vi "LM3Sxxxx_Timer_Config.vi"(8 "error in (no error)":errorcluster, 10 "Config Data":string[](array[string]), 11 "Interrupt Name":string) -> (0 "error out":errorcluster, 3 "Interrupt Configuration":string[](array[string]))   [LabVIEW 2011]
panel:
  in  "Trigger":u32(ring) items=["Rising edge"=0, "Falling edge"=1028, "Both edges"=3084]
  in  "Trigger":u32(ring) items=["Rising edge"=0, "Falling edge"=1028]
  in  "Units":u32(ring)=1 items=["Milliseconds"=1, "Microseconds"=2, "Ticks"=0]
  in  "Count":u16=1000
  in  "Count":u16=1000
  in  "Period":u32=1000
  in  "edge capture":bool
  in  "timer capture":bool
  in  "timer":bool=TRUE
  in  "help":bool
  in  "cancel":bool
  in  "ok":bool
  # "Mode"
  # "32-bit Timer"
  # "16-bit Timer Capture"
  # "16-bit Edge Counter"
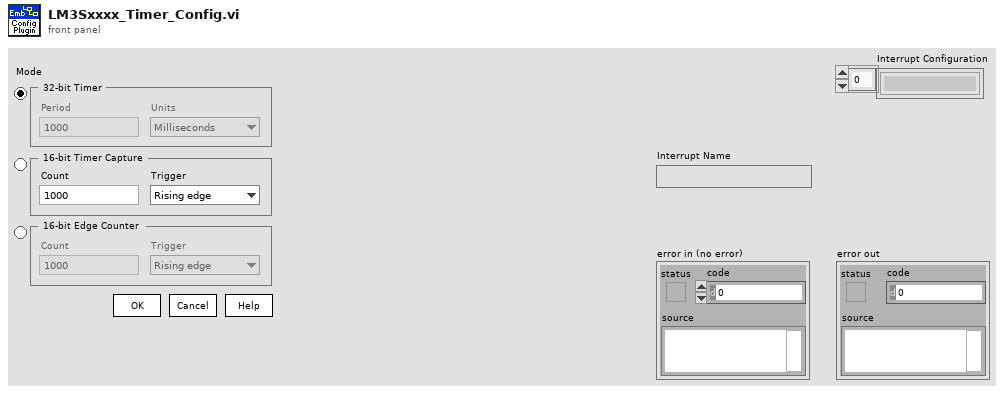
[diagram p1: front panel]
types:
  T1 = enum8{"Enabled", "Disabled", "Disabled and Grayed Out"}
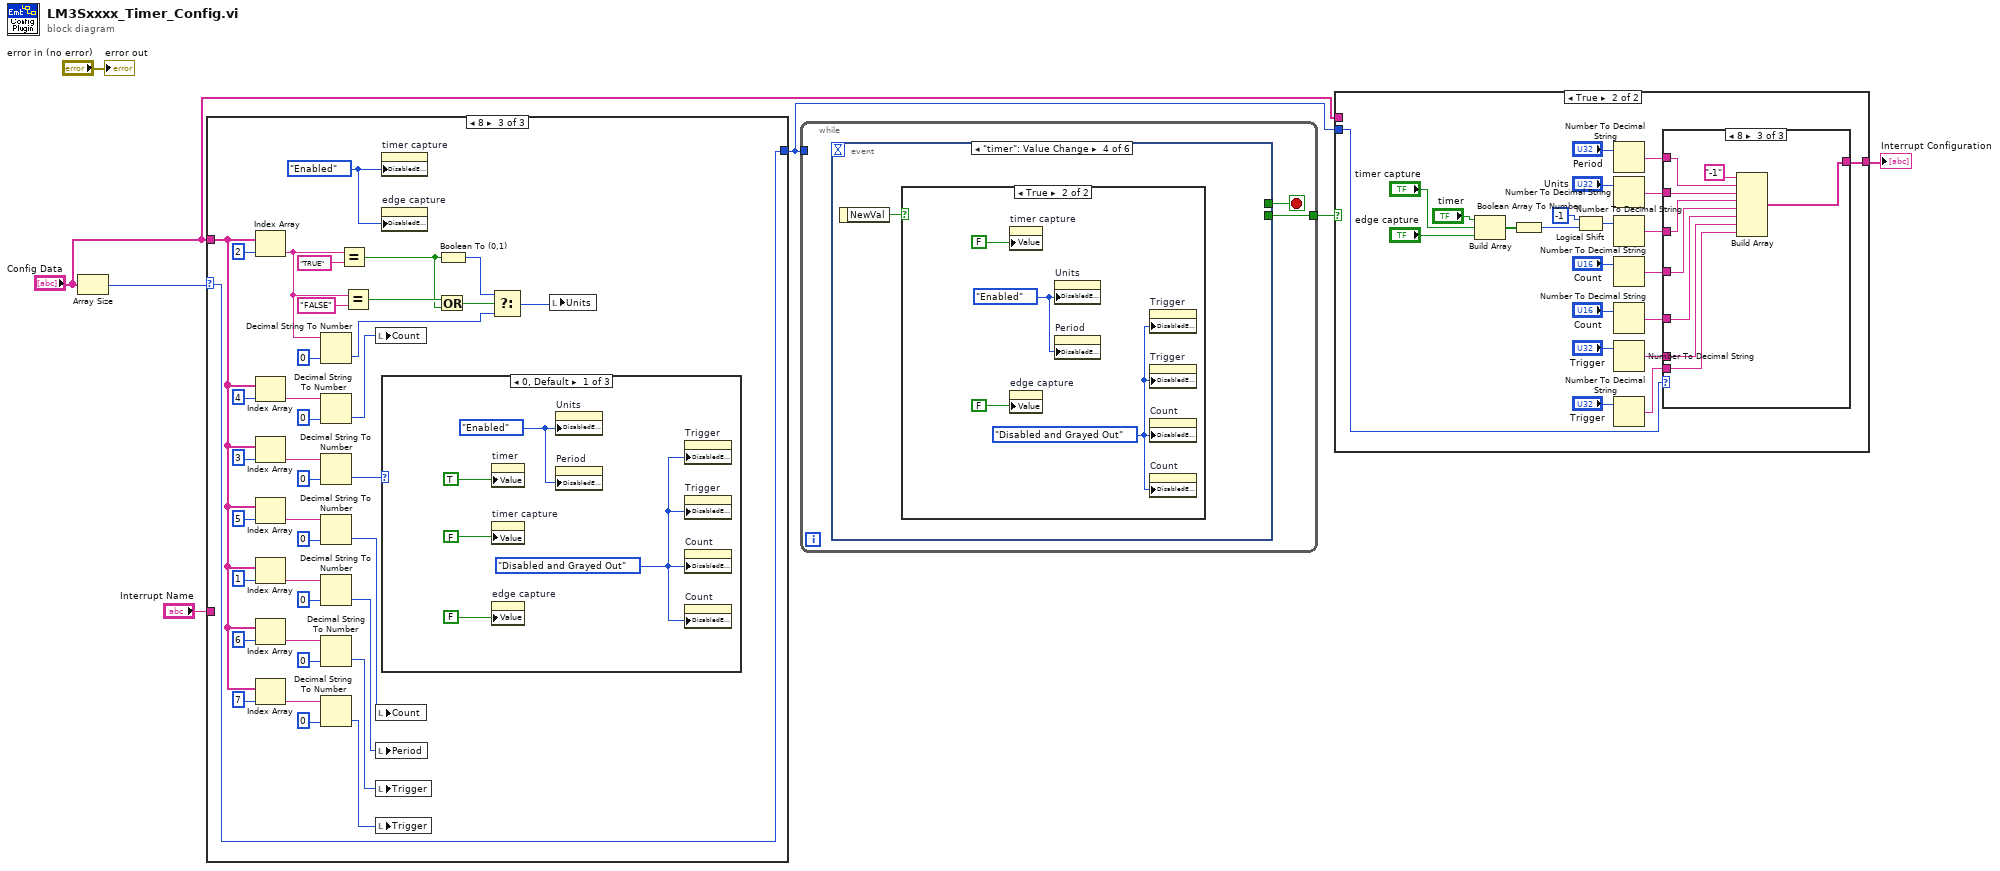
[diagram p0: block diagram]
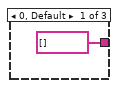
[diagram p3: hidden frame]
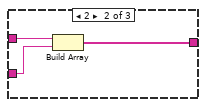
[diagram p4: hidden frame]
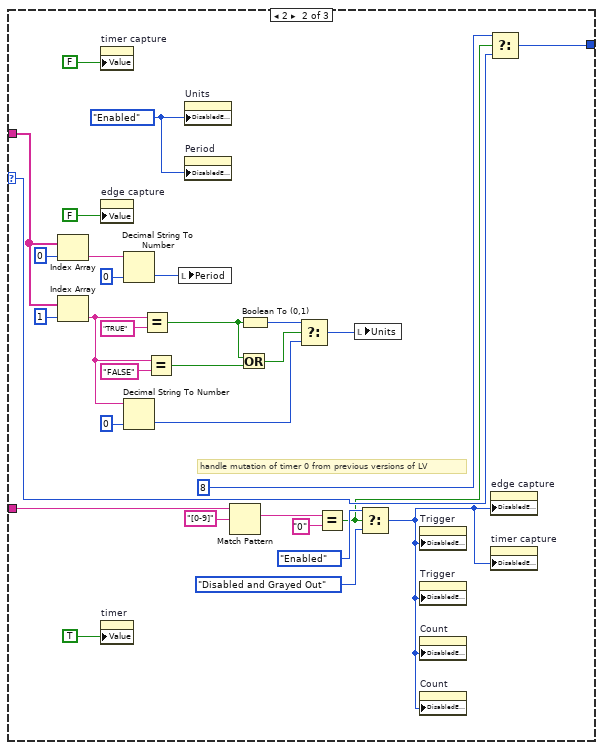
[diagram p6: hidden frame]
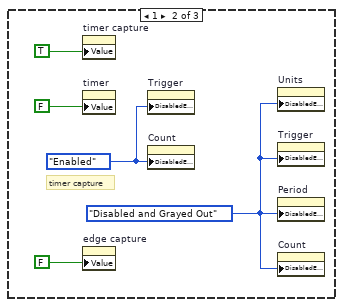
[diagram p7: hidden frame]
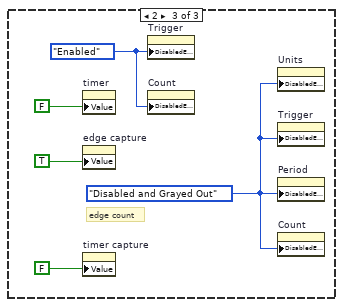
[diagram p8: hidden frame]
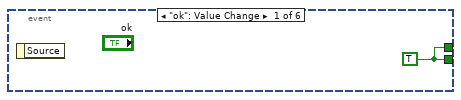
[diagram p9: hidden frame]
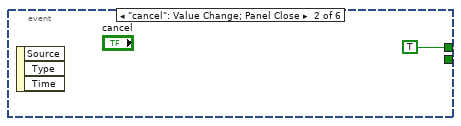
[diagram p10: hidden frame]
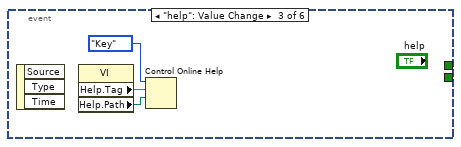
[diagram p11: hidden frame]
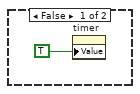
[diagram p12: hidden frame]
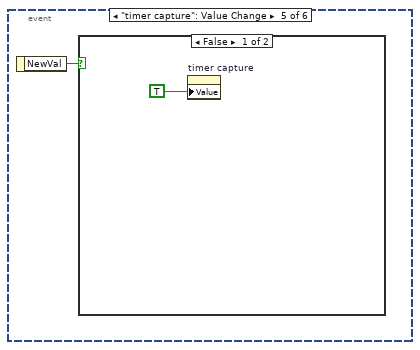
[diagram p13: hidden frame]
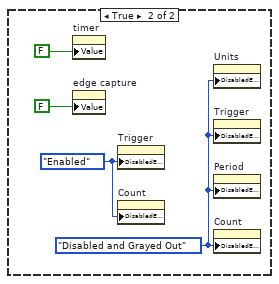
[diagram p14: hidden frame]
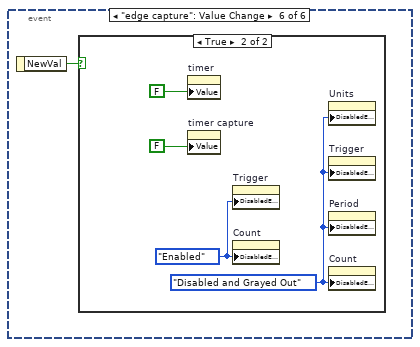
[diagram p15: hidden frame]
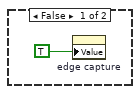
[diagram p16: hidden frame]
diagram:
  n1 = Array Size(array="Config Data") -> (size(s)=w3:i32)
  n2 = case shown="8" w3 {
    selector: w3 -> [w8 w23 w77]
    tunnel: "Config Data" -> [_ w39 w62]
    tunnel: [w8 w22 w77] -> w1
    tunnel: "Interrupt Name" -> [_ w27 _]
    frame Default {
    }
    frame 2 {
      w29 = T1."Enabled" ("Disabled")
      # "handle mutation of timer 0 from previous versions of LV"
      n3 = Index Array(array=w39, index=0) -> (element=w35:string)
      n4 = Index Array(array=w39, index=1) -> (element=w15:string)
      n5 = property on="timer capture" class="Bool (strict)"("Value"=FALSE ("timer capture")) -> ()  [unwired: 2 in, 2 out]
      n6 = property on="edge capture" class="Bool (strict)"("Value"=FALSE ("edge capture")) -> ()  [unwired: 2 in, 2 out]
      n7 = property on="timer" class="Bool (strict)"("Value"=TRUE ("timer")) -> ()  [unwired: 2 in, 2 out]
      n8 = Decimal String To Number(string=w35, default (0L)=u32 0) -> (number=w34:u32)  [unwired: 1 in, 1 out]
      n9 = Decimal String To Number(string=w15, default (0L)=u32 0) -> (number=w11:u32)  [unwired: 1 in, 1 out]
      n10 = Equal?(x=w15, y="TRUE") -> (x = y?=w14:bool)
      n11 = Equal?(x=w15, y="FALSE") -> (x = y?=w13:bool)
      n12 = local write "Period"(w34) -> ()
      n13 = property on="Units" class="Ring (strict)"("DisabledEnum"=w29) -> ()  [unwired: 2 in, 2 out]
      n14 = property on="Period" class="DigNum (strict)"("DisabledEnum"=w29) -> ()  [unwired: 2 in, 2 out]
      n15 = Match Pattern(string=w27, regular expression="[0-9]") -> (match substring=w20:string)  [unwired: 1 in, 3 out]
      n16 = Or(x=w14, y=w13) -> (x .or. y?=w12:bool)
      n17 = Boolean To (0,1)(Boolean=w14) -> (0, 1=w10:i16)
      n18 = Select(t=w10, s=w12, f=w11) -> (s? t:f=w9:u32)
      n19 = Equal?(x=w20, y="0") -> (x = y?=w19:bool)
      n20 = local write "Units"(w9) -> ()
      n21 = Select(t=T1."Enabled", s=w19, f=T1."Disabled and Grayed Out" ("Disabled")) -> (s? t:f=w25:T1)
      n22 = property on="Trigger" class="Ring (strict)"("DisabledEnum"=w25) -> ()  [unwired: 2 in, 2 out]
      n23 = property on="Trigger" class="Ring (strict)"("DisabledEnum"=w25) -> ()  [unwired: 2 in, 2 out]
      n24 = property on="Count" class="DigNum (strict)"("DisabledEnum"=w25) -> ()  [unwired: 2 in, 2 out]
      n25 = property on="Count" class="DigNum (strict)"("DisabledEnum"=w25) -> ()  [unwired: 2 in, 2 out]
      n26 = Select(t=8, s=w19, f=w23) -> (s? t:f=w22:i32)
      n27 = property on="edge capture" class="Bool (strict)"("DisabledEnum"=w25) -> ()  [unwired: 2 in, 2 out]
      n28 = property on="timer capture" class="Bool (strict)"("DisabledEnum"=w25) -> ()  [unwired: 2 in, 2 out]
    }
    frame 8 {
      w49 = T1."Enabled" ("Disabled")
      n29 = Index Array(array=w62, index=2) -> (element=w44:string)
      n30 = Index Array(array=w62, index=4) -> (element=w60:string)
      n31 = Index Array(array=w62, index=3) -> (element=w66:string)
      n32 = Index Array(array=w62, index=5) -> (element=w57:string)
      n33 = Index Array(array=w62, index=1) -> (element=w75:string)
      n34 = Index Array(array=w62, index=6) -> (element=w53:string)
      n35 = Index Array(array=w62, index=7) -> (element=w52:string)
      n36 = Decimal String To Number(string=w44, default (0L)=u32 0) -> (number=w41:u32)  [unwired: 1 in, 1 out]
      n37 = Decimal String To Number(string=w60, default (0L)=u16 0) -> (number=w59:u16)  [unwired: 1 in, 1 out]
      n38 = Decimal String To Number(string=w66, default (0L)=u32 0) -> (number=w65:u32)  [unwired: 1 in, 1 out]
      n39 = Decimal String To Number(string=w57, default (0L)=u16 0) -> (number=w56:u16)  [unwired: 1 in, 1 out]
      n40 = Decimal String To Number(string=w75, default (0L)=u32 0) -> (number=w71:u32)  [unwired: 1 in, 1 out]
      n41 = Decimal String To Number(string=w53, default (0L)=u32 0) -> (number=w51:u32)  [unwired: 1 in, 1 out]
      n42 = Decimal String To Number(string=w52, default (0L)=u32 0) -> (number=w50:u32)  [unwired: 1 in, 1 out]
      n43 = Equal?(x=w44, y="TRUE") -> (x = y?=w46:bool)
      n44 = Equal?(x=w44, y="FALSE") -> (x = y?=w47:bool)
      n45 = local write "Count"(w59) -> ()
      n46 = local write "Count"(w56) -> ()
      n47 = local write "Period"(w71) -> ()
      n48 = local write "Trigger"(w51) -> ()
      n49 = local write "Trigger"(w50) -> ()
      n50 = property on="timer capture" class="Bool (strict)"("DisabledEnum"=w49) -> ()  [unwired: 2 in, 2 out]
      n51 = property on="edge capture" class="Bool (strict)"("DisabledEnum"=w49) -> ()  [unwired: 2 in, 2 out]
      n52 = case shown="0, Default" w65 {
        frame 0, Default {
          w78 = T1."Disabled and Grayed Out" ("Disabled")
          w79 = T1."Enabled" ("Disabled")
          n53 = property on="timer" class="Bool (strict)"("Value"=TRUE ("timer")) -> ()  [unwired: 2 in, 2 out]
          n54 = property on="timer capture" class="Bool (strict)"("Value"=FALSE ("timer capture")) -> ()  [unwired: 2 in, 2 out]
          n55 = property on="edge capture" class="Bool (strict)"("Value"=FALSE ("edge capture")) -> ()  [unwired: 2 in, 2 out]
          n56 = property on="Units" class="Ring (strict)"("DisabledEnum"=w79) -> ()  [unwired: 2 in, 2 out]
          n57 = property on="Period" class="DigNum (strict)"("DisabledEnum"=w79) -> ()  [unwired: 2 in, 2 out]
          n58 = property on="Trigger" class="Ring (strict)"("DisabledEnum"=w78) -> ()  [unwired: 2 in, 2 out]
          n59 = property on="Trigger" class="Ring (strict)"("DisabledEnum"=w78) -> ()  [unwired: 2 in, 2 out]
          n60 = property on="Count" class="DigNum (strict)"("DisabledEnum"=w78) -> ()  [unwired: 2 in, 2 out]
          n61 = property on="Count" class="DigNum (strict)"("DisabledEnum"=w78) -> ()  [unwired: 2 in, 2 out]
        }
        frame 1 {
          w84 = T1."Enabled" ("Disabled")
          w83 = T1."Disabled and Grayed Out" ("Disabled")
          # "timer capture"
          n62 = property on="timer capture" class="Bool (strict)"("Value"=TRUE ("timer capture")) -> ()  [unwired: 2 in, 2 out]
          n63 = property on="timer" class="Bool (strict)"("Value"=FALSE ("timer")) -> ()  [unwired: 2 in, 2 out]
          n64 = property on="edge capture" class="Bool (strict)"("Value"=FALSE ("edge capture")) -> ()  [unwired: 2 in, 2 out]
          n65 = property on="Trigger" class="Ring (strict)"("DisabledEnum"=w84) -> ()  [unwired: 2 in, 2 out]
          n66 = property on="Count" class="DigNum (strict)"("DisabledEnum"=w84) -> ()  [unwired: 2 in, 2 out]
          n67 = property on="Units" class="Ring (strict)"("DisabledEnum"=w83) -> ()  [unwired: 2 in, 2 out]
          n68 = property on="Trigger" class="Ring (strict)"("DisabledEnum"=w83) -> ()  [unwired: 2 in, 2 out]
          n69 = property on="Period" class="DigNum (strict)"("DisabledEnum"=w83) -> ()  [unwired: 2 in, 2 out]
          n70 = property on="Count" class="DigNum (strict)"("DisabledEnum"=w83) -> ()  [unwired: 2 in, 2 out]
        }
        frame 2 {
          w88 = T1."Enabled" ("Disabled")
          w89 = T1."Disabled and Grayed Out" ("Disabled")
          # "edge count"
          n71 = property on="timer" class="Bool (strict)"("Value"=FALSE ("timer")) -> ()  [unwired: 2 in, 2 out]
          n72 = property on="edge capture" class="Bool (strict)"("Value"=TRUE ("edge capture")) -> ()  [unwired: 2 in, 2 out]
          n73 = property on="timer capture" class="Bool (strict)"("Value"=FALSE ("timer capture")) -> ()  [unwired: 2 in, 2 out]
          n74 = property on="Trigger" class="Ring (strict)"("DisabledEnum"=w88) -> ()  [unwired: 2 in, 2 out]
          n75 = property on="Count" class="DigNum (strict)"("DisabledEnum"=w88) -> ()  [unwired: 2 in, 2 out]
          n76 = property on="Units" class="Ring (strict)"("DisabledEnum"=w89) -> ()  [unwired: 2 in, 2 out]
          n77 = property on="Trigger" class="Ring (strict)"("DisabledEnum"=w89) -> ()  [unwired: 2 in, 2 out]
          n78 = property on="Period" class="DigNum (strict)"("DisabledEnum"=w89) -> ()  [unwired: 2 in, 2 out]
          n79 = property on="Count" class="DigNum (strict)"("DisabledEnum"=w89) -> ()  [unwired: 2 in, 2 out]
        }
      }
      n80 = Or(x=w47, y=w46) -> (x .or. y?=w45:bool)
      n81 = Boolean To (0,1)(Boolean=w46) -> (0, 1=w42:i16)
      n82 = Select(t=w42, s=w45, f=w41) -> (s? t:f=w40:u32)
      n83 = local write "Units"(w40) -> ()
    }
  }
  n84 = while {
    tunnel: [w93] -> w6
    tunnel: w1 -> [_]
    stop <- w94 stop-if-true
    n85 = event shown="[3] \"timer\": Value Change" {
      selector: _ -> [_ _ _ _ _ _]
      dyn-events: _ -> [_ _ _ _ _ _]
      timeout: _ -> [_ _ _ _ _ _]
      tunnel: [w95 TRUE _ _ _ _] -> w94
      tunnel: [w95 _ _ _ _ _] -> w93
      event "ok": Value Change {
        w95 = TRUE
        n86 = event-data() -> ()  [unwired: 2 out]
      }
      event "cancel": Value Change; Panel Close {
        n87 = event-data() -> ()  [unwired: 4 out]
      }
      event "help": Value Change {
        n88 = event-data() -> ()  [unwired: 4 out]
        n89 = property class="VI"() -> ("Help.Tag"=w97:string, "Help.Path"=w98:path)  [unwired: 2 in, 2 out]
        n90 = Control Online Help(2:w98, 3:w97, 4:enum16{"Contents", "Key", "Close"}."Key" ("Operation")) -> ()  [unwired: 1 in, 1 out]
      }
      event "timer": Value Change {
        n91 = event-data() -> ("NewVal"=w100:bool)  [unwired: 1 out]
        n92 = case shown="True" w100 {
          frame False {
            n93 = property on="timer" class="Bool (strict)"("Value"=TRUE ("timer")) -> ()  [unwired: 2 in, 2 out]
          }
          frame True {
            w105 = T1."Disabled and Grayed Out" ("Disabled")
            w104 = T1."Enabled" ("Disabled")
            n94 = property on="timer capture" class="Bool (strict)"("Value"=FALSE ("timer capture")) -> ()  [unwired: 2 in, 2 out]
            n95 = property on="edge capture" class="Bool (strict)"("Value"=FALSE ("edge capture")) -> ()  [unwired: 2 in, 2 out]
            n96 = property on="Units" class="Ring (strict)"("DisabledEnum"=w104) -> ()  [unwired: 2 in, 2 out]
            n97 = property on="Period" class="DigNum (strict)"("DisabledEnum"=w104) -> ()  [unwired: 2 in, 2 out]
            n98 = property on="Trigger" class="Ring (strict)"("DisabledEnum"=w105) -> ()  [unwired: 2 in, 2 out]
            n99 = property on="Trigger" class="Ring (strict)"("DisabledEnum"=w105) -> ()  [unwired: 2 in, 2 out]
            n100 = property on="Count" class="DigNum (strict)"("DisabledEnum"=w105) -> ()  [unwired: 2 in, 2 out]
            n101 = property on="Count" class="DigNum (strict)"("DisabledEnum"=w105) -> ()  [unwired: 2 in, 2 out]
          }
        }
      }
      event "timer capture": Value Change {
        n102 = event-data() -> ("NewVal"=w106:bool)  [unwired: 1 out]
        n103 = case shown="False" w106 {
          frame False {
            n104 = property on="timer capture" class="Bool (strict)"("Value"=TRUE ("timer capture")) -> ()  [unwired: 2 in, 2 out]
          }
          frame True {
            w108 = T1."Enabled" ("Disabled")
            w109 = T1."Disabled and Grayed Out" ("Disabled")
            n105 = property on="timer" class="Bool (strict)"("Value"=FALSE ("timer")) -> ()  [unwired: 2 in, 2 out]
            n106 = property on="edge capture" class="Bool (strict)"("Value"=FALSE ("edge capture")) -> ()  [unwired: 2 in, 2 out]
            n107 = property on="Trigger" class="Ring (strict)"("DisabledEnum"=w108) -> ()  [unwired: 2 in, 2 out]
            n108 = property on="Count" class="DigNum (strict)"("DisabledEnum"=w108) -> ()  [unwired: 2 in, 2 out]
            n109 = property on="Units" class="Ring (strict)"("DisabledEnum"=w109) -> ()  [unwired: 2 in, 2 out]
            n110 = property on="Trigger" class="Ring (strict)"("DisabledEnum"=w109) -> ()  [unwired: 2 in, 2 out]
            n111 = property on="Period" class="DigNum (strict)"("DisabledEnum"=w109) -> ()  [unwired: 2 in, 2 out]
            n112 = property on="Count" class="DigNum (strict)"("DisabledEnum"=w109) -> ()  [unwired: 2 in, 2 out]
          }
        }
      }
      event "edge capture": Value Change {
        n113 = event-data() -> ("NewVal"=w112:bool)  [unwired: 1 out]
        n114 = case shown="True" w112 {
          frame False {
            n115 = property on="edge capture" class="Bool (strict)"("Value"=TRUE ("edge capture")) -> ()  [unwired: 2 in, 2 out]
          }
          frame True {
            w114 = T1."Disabled and Grayed Out" ("Disabled")
            w115 = T1."Enabled" ("Disabled")
            n116 = property on="timer" class="Bool (strict)"("Value"=FALSE ("timer")) -> ()  [unwired: 2 in, 2 out]
            n117 = property on="timer capture" class="Bool (strict)"("Value"=FALSE ("timer capture")) -> ()  [unwired: 2 in, 2 out]
            n118 = property on="Trigger" class="Ring (strict)"("DisabledEnum"=w115) -> ()  [unwired: 2 in, 2 out]
            n119 = property on="Count" class="DigNum (strict)"("DisabledEnum"=w115) -> ()  [unwired: 2 in, 2 out]
            n120 = property on="Units" class="Ring (strict)"("DisabledEnum"=w114) -> ()  [unwired: 2 in, 2 out]
            n121 = property on="Trigger" class="Ring (strict)"("DisabledEnum"=w114) -> ()  [unwired: 2 in, 2 out]
            n122 = property on="Period" class="DigNum (strict)"("DisabledEnum"=w114) -> ()  [unwired: 2 in, 2 out]
            n123 = property on="Count" class="DigNum (strict)"("DisabledEnum"=w114) -> ()  [unwired: 2 in, 2 out]
          }
        }
      }
    }
  }
  n124 = case shown="True" w6 {
    tunnel: "Config Data" -> [w118 _]
    tunnel: [w118 w137] -> w4
    tunnel: w1 -> [_ w140]
    frame False {
    }
    frame True {
      n125 = Build Array("timer", "timer capture", "edge capture") -> (w133:bool[])
      n126 = Boolean Array To Number(Boolean array=w133) -> (number=w132:u32)
      n127 = Logical Shift(y=i8 -1, x=w132) -> (x << y=w130:u32)
      n128 = Number To Decimal String(number="Period") -> (decimal integer string=w138:string)  [unwired: 1 in]
      n129 = Number To Decimal String(number="Units") -> (decimal integer string=w119:string)  [unwired: 1 in]
      n130 = Number To Decimal String(number=w130) -> (decimal integer string=w129:string)  [unwired: 1 in]
      n131 = Number To Decimal String(number="Count") -> (decimal integer string=w127:string)  [unwired: 1 in]
      n132 = Number To Decimal String(number="Count") -> (decimal integer string=w125:string)  [unwired: 1 in]
      n133 = Number To Decimal String(number="Trigger") -> (decimal integer string=w123:string)  [unwired: 1 in]
      n134 = Number To Decimal String(number="Trigger") -> (decimal integer string=w121:string)  [unwired: 1 in]
      n135 = case shown="8" w140 {
        tunnel: w138 -> [_ w144 w153]
        tunnel: w119 -> [_ w143 w152]
        tunnel: [string[] [] w142 w151] -> w137
        tunnel: w129 -> [_ _ w150]
        tunnel: w127 -> [_ _ w149]
        tunnel: w125 -> [_ _ w148]
        tunnel: w123 -> [_ _ w147]
        tunnel: w121 -> [_ _ w146]
        frame 0, Default {
        }
        frame 2 {
          n136 = Build Array(w144, w143) -> (w142:string[])
        }
        frame 8 {
          n137 = Build Array("-1" ("element"), w153, w152, w150, w149, w148, w147, w146) -> (w151:string[])
        }
      }
    }
  }
  "Interrupt Configuration" <- w4
  "error out" <- "error in (no error)"
